vi "Write Waveform.vi"(8 "error in (no error)":errorcluster, 10 "Waveform":waveform(dbl)[](array[waveform]), 11 "AI_Task in":refnum<class "AI_Task.lvclass">) -> (0 "error out":errorcluster, 3 "AI_Task out":refnum<class "AI_Task.lvclass">)   [LabVIEW 2025, in "AI_Task.lvlib" / "AI_Task.lvclass"]
uses:
  AI_Task.lvclass
  AI_Task.lvclass/AI_Task.ctl
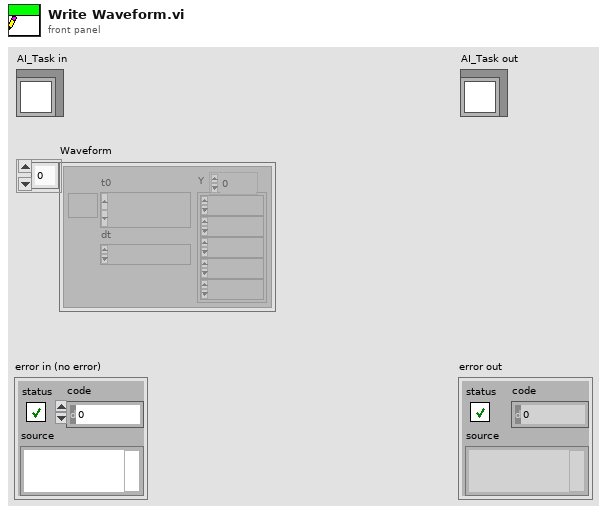
[diagram p1: front panel]
types:
  T1 = typedef "Task_Abstr.lvlib/Task_Abstr.lvclass/DataContainer.ctl" = map{string, T2}
  T2 = typedef "Task_Abstr.lvlib/Task_Abstr.lvclass/WaveformData.ctl" = cluster{"StartTime":timestamp, "StopTime":timestamp, "Waveform":waveform(dbl)[]}
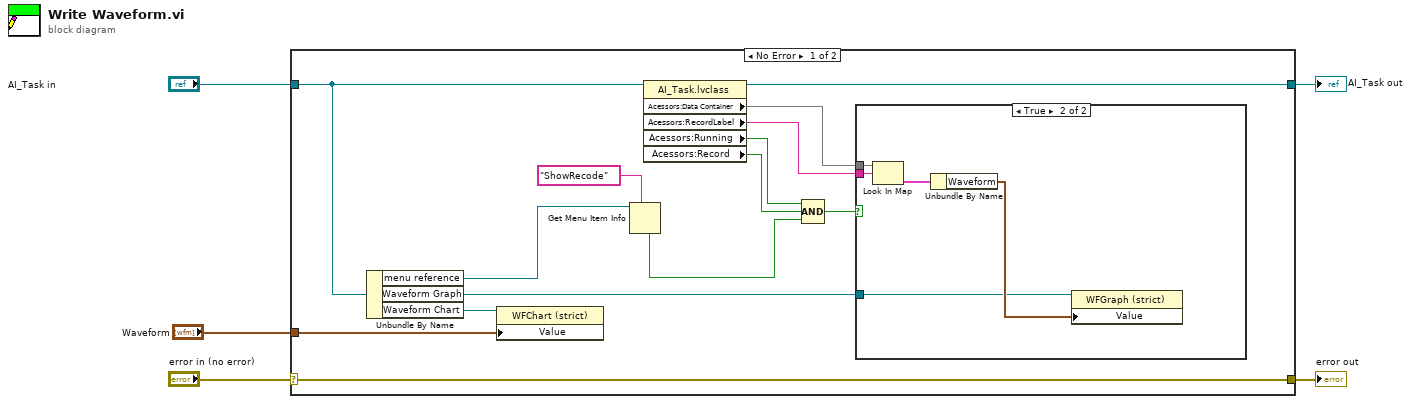
[diagram p0: block diagram]
diagram:
  n1 = case shown="No Error" "error in (no error)" {
    selector: "error in (no error)" -> [w19 w25]
    tunnel: [w19 w25] -> w4
    tunnel: [w15 w26] -> w2
    tunnel: "AI_Task in" -> [w18 w26]
    tunnel: "Waveform" -> [w16 _]
    frame No Error {
      n2 = Unbundle By Name(w18) -> ("menu reference"=w9:refnum<k9>, "Waveform Graph"=w12:refnum<vi>, "Waveform Chart"=w17:refnum<vi>)
      n3 = property class="WFChart (strict)"(reference=w17, "Value"=w16) -> ()  [unwired: 1 in, 2 out]
      n4 = Get Menu Item Info(7:"ShowRecode" ("item tag"), 11:w9) -> (4:w7:bool)  [unwired: 1 in, 6 out]
      n5 = property class="AI_Task.lvclass"(reference=w18) -> (reference out=w15:refnum<class "AI_Task.lvclass">, "Acessors:Data Container"=w14:T1, "Acessors:RecordLabel"=w13:string, "Acessors:Running"=w11:bool, "Acessors:Record"=w10:bool)  [unwired: 1 in, 1 out]
      n6 = Compound Arithmetic op=AND(w11, w10, w7) -> (w6:bool)
      n7 = case shown="True" w6 {
        tunnel: w14 -> [_ w24]
        tunnel: w13 -> [_ w23]
        tunnel: w12 -> [_ w20]
        frame False {
        }
        frame True {
          n8 = Look In Map(map=w24, key=w23) -> (value=w22:T2)  [unwired: 1 in, 1 out]
          n9 = Unbundle By Name(w22) -> ("Waveform"=w21:waveform(dbl)[])
          n10 = property class="WFGraph (strict)"(reference=w20, "Value"=w21) -> ()  [unwired: 1 in, 2 out]
        }
      }
    }
    frame Error {
    }
  }
  "error out" <- w4
  "AI_Task out" <- w2
